vi "TSL_Busy_Check.vi"(8 "error in (no error)":errorcluster, 10 "Wait time(msec)":i32, 11 ".NET Reference in":refnum<k24>) -> (0 "error out":errorcluster, 3 "Reference out":refnum<k24>)   [LabVIEW 2017]
uses:
  C:/Users/Ssantec_Test/Documents/Instrument_DLL_Sample_Labview_20250826_Ver1.5.0_x64/DLL/InstrumentDLL.dll
  DLL/InstrumentDLL.dll
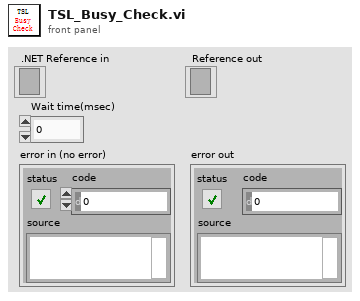
[diagram p1: front panel]
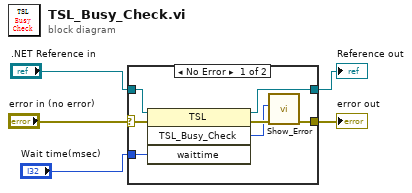
[diagram p0: block diagram]
diagram:
  n1 = case shown="No Error" "error in (no error)" {
    selector: "error in (no error)" -> [w9 w13]
    tunnel: "Wait time(msec)" -> [w12 _]
    tunnel: ".NET Reference in" -> [w11 w14]
    tunnel: [w10 w14] -> w3
    tunnel: [w6 w13] -> w1
    frame No Error {
      n2 = invoke on="调用节点" class="TSL" method="TSL_Busy_Check"(reference=w11, error in=w9, "waittime"=w12) -> (reference out=w10:refnum<k24>, error out=w8:errorcluster, "TSL_Busy_Check"=w7:i32)  [unwired: 1 in, 1 out]
      n3 = call "Show_Error.vi"("error in (no error)"=w8, "Error"=w7) -> ("error out"=w6:errorcluster)  [unwired: 9 in]
    }
    frame Error {
    }
  }
  "Reference out" <- w3
  "error out" <- w1
